vi "XML string.vi"(8 "tag":string, 11 "String":string) -> (0 "Tag Found":bool, 3 "string":string)   [LabVIEW 2013]
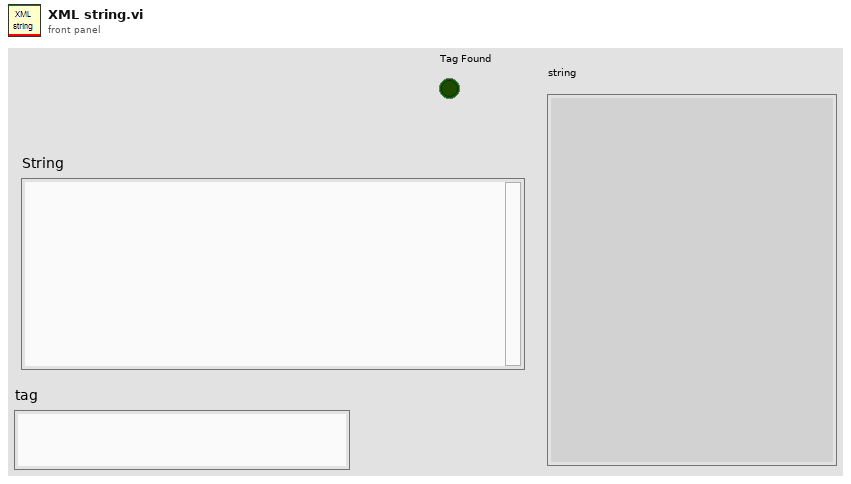
[diagram p1: front panel]
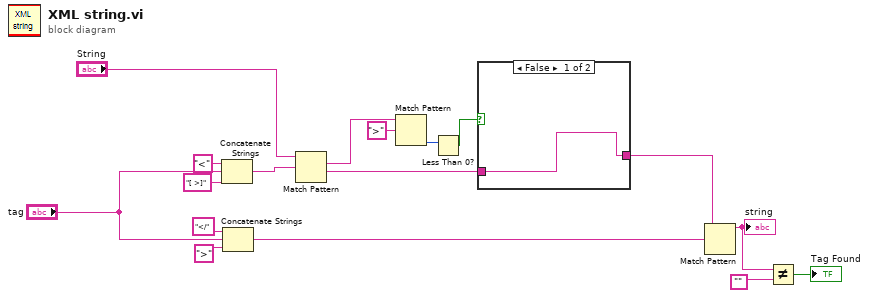
[diagram p0: block diagram]
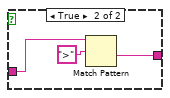
[diagram p2: hidden frame]
diagram:
  n1 = Concatenate Strings("<" ("string"), "tag", "[ >]" ("string")) -> (w15:string)
  n2 = Concatenate Strings("</" ("string"), "tag", ">" ("string")) -> (w14:string)
  n3 = Match Pattern(string="String", regular expression=w15) -> (match substring=w9:string, after substring=w5:string)  [unwired: 1 in, 2 out]
  n4 = Match Pattern(string=w9, regular expression=">") -> (offset past match=w7:i32)  [unwired: 1 in, 3 out]
  n5 = Less Than 0?(x=w7) -> (x < 0?=w6:bool)
  n6 = case shown="False" w6 {
    tunnel: w5 -> [w18 w20]
    tunnel: [w18 w19] -> w4
    frame False {
    }
    frame True {
      n7 = Match Pattern(string=w20, regular expression=">") -> (after substring=w19:string)  [unwired: 1 in, 3 out]
    }
  }
  n8 = Match Pattern(string=w4, regular expression=w14) -> (before substring=w3:string)  [unwired: 1 in, 3 out]
  "string" <- w3
  n9 = Not Equal?(x=w3, y="") -> (x != y?=→"Tag Found":bool)
